vi "set_iterations_per_pixel.vi"(8 "error in (no error)":errorcluster, 10 "iterations per pixel":i32, 11 "FPGAWrapperDL090211Galvo in":refnum<class "FPGAWrapperDL090211Galvo.lvclass">) -> (0 "error out":errorcluster, 3 "FPGAWrapperDL090211Galvo out":refnum<class "FPGAWrapperDL090211Galvo.lvclass">)   [LabVIEW 2010, in "FPGAWrapperDL090211Galvo.lvclass"]
uses:
  FPGAWrapperDL090211Galvo.lvclass
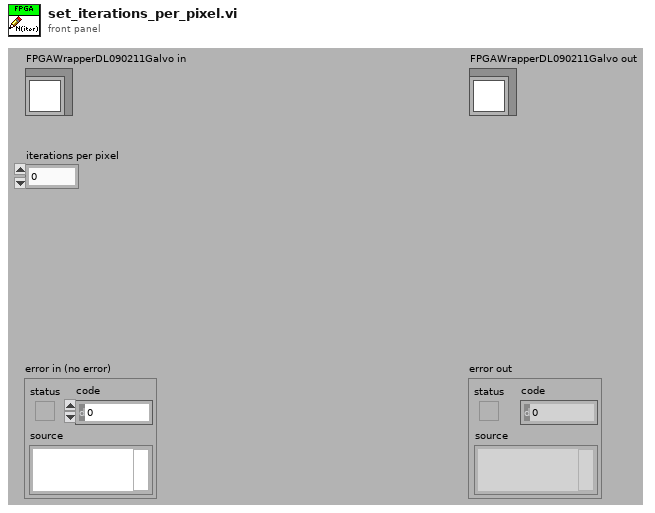
[diagram p1: front panel]
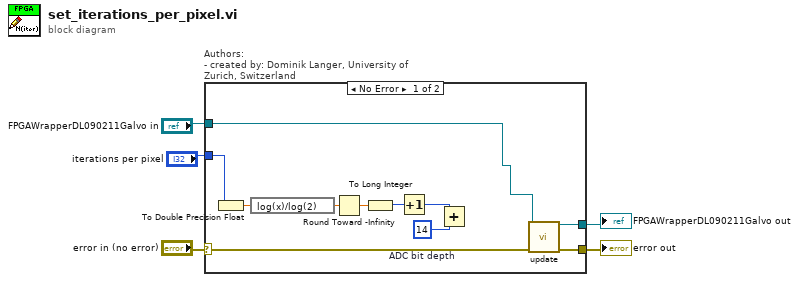
[diagram p0: block diagram]
diagram:
  n1 = case "Authors: \n- created by: Dominik Langer, University of Zurich, Switzerland" shown="No Error" "error in (no error)" {
    selector: "error in (no error)" -> [w9 w17]
    tunnel: "FPGAWrapperDL090211Galvo in" -> [w6 w18]
    tunnel: [w8 w18] -> w1
    tunnel: [w7 w17] -> w2
    tunnel: "iterations per pixel" -> [w10 _]
    frame No Error {
      w15 = 14  # ADC bit depth
      n2 = To Double Precision Float(number=w10) -> (double precision float=w12:dbl)
      n3 = expression code="log(x)/log(2)"(w12) -> (w11:dbl)
      n4 = Round Toward -Infinity(1:w11) -> (0:w16:dbl)
      n5 = To Long Integer(number=w16) -> (32bit integer=w14:i32)
      n6 = Increment(x=w14) -> (x+1=w13:i32)
      n7 = Add(x=w13, y=w15) -> ()  [unwired: 1 out]
      n8 = call-dynamic "update.vi"("error in (no error)"=w9, "FPGAWrapperDL120115Galvo in"=w6) -> ("error out"=w7:errorcluster, "FPGAWrapperDL120115Galvo out"=w8:refnum<class "FPGAWrapperDL090211Galvo.lvclass">)  [unwired: 8 in]
    }
    frame Error {
    }
  }
  "error out" <- w2
  "FPGAWrapperDL090211Galvo out" <- w1
